vi "ResMgr-Request ExitEvent.vi"(6 "Timeout In ms (5000 ms)":i32=5000, 7 "WatchDogQ":refnum<queue>, 8 "Error In":errorcluster caption="error in (no error)") -> (0 "error out":errorcluster, 3 "CSMExit":refnum<user-event>)   [LabVIEW 2017, in "Communicable State Machine.lvlib"]
uses:
  Communicable State Machine.lvlib
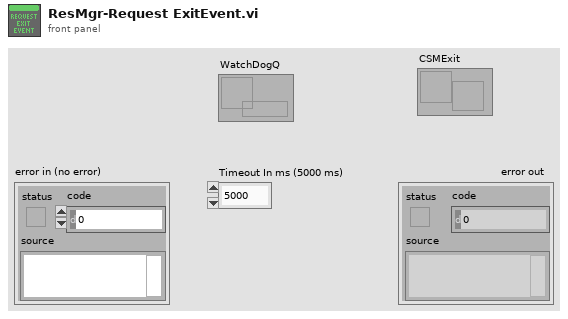
[diagram p1: front panel]
types:
  T1 = cluster{"ResType":string, "RespQ":refnum<queue>, "Parameter":string, "WatchDogQ":refnum<queue>}
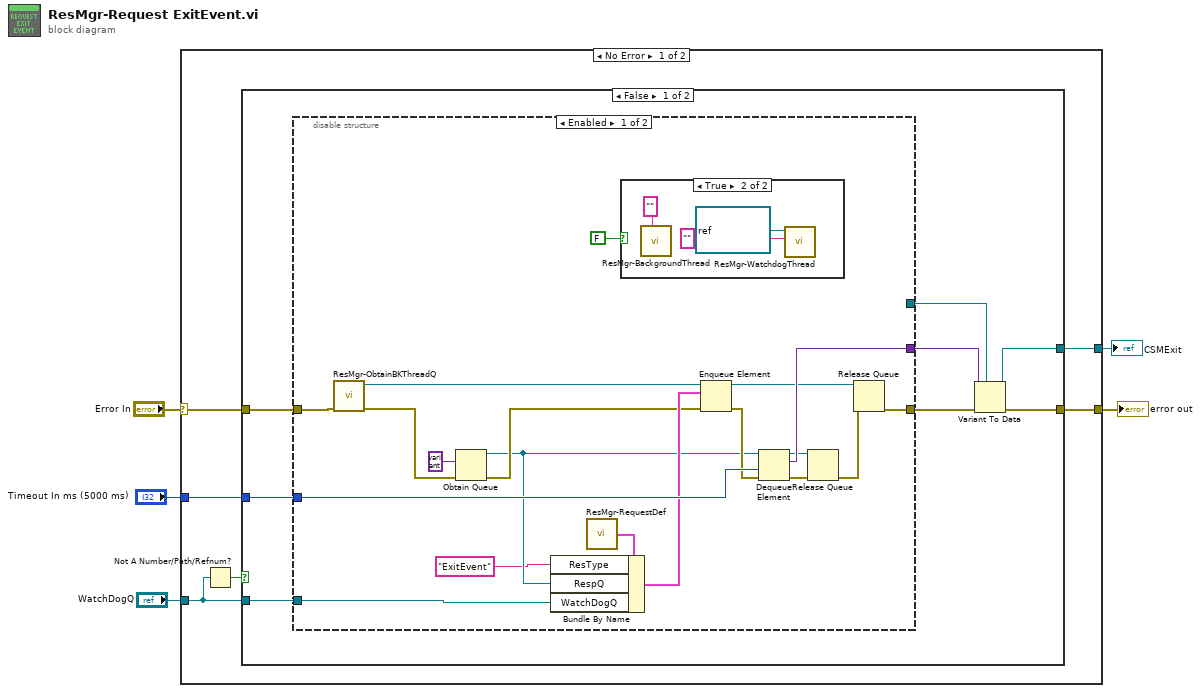
[diagram p0: block diagram]
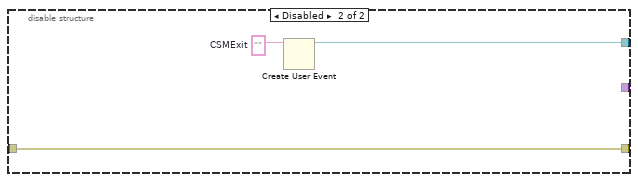
[diagram p3: hidden frame]
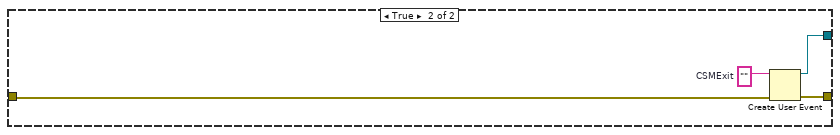
[diagram p4: hidden frame]
diagram:
  n1 = case shown="No Error" "Error In" {
    selector: "Error In" -> [w10 w49]
    tunnel: [w9 w49] -> w5
    tunnel: [w8 _] -> w1
    tunnel: "Timeout In ms (5000 ms)" -> [w11 _]
    tunnel: "WatchDogQ" -> [w7 _]
    frame No Error {
      n2 = Not A Number/Path/Refnum?(number/path/refnum=w7) -> (NaN/Path/Refnum?=w6:bool)
      n3 = case shown="False" w6 {
        tunnel: w11 -> [w18 _]
        tunnel: w10 -> [w17 w45]
        tunnel: w7 -> [w16 _]
        tunnel: [w15 w47] -> w9
        tunnel: [w12 w46] -> w8
        frame False {
          n4 = disable-structure shown="Enabled" {
            disable-tunnel: [w38 w44] -> w19
            disable-tunnel: w18 -> [w37 _]
            disable-tunnel: [w36 _] -> w14
            disable-tunnel: w17 -> [w21 w44]
            disable-tunnel: w16 -> [w25 _]
            disable-tunnel: [_ w42] -> w13
            frame Enabled {
              n5 = call "ResMgr-ObtainBKThreadQ.vi"("error in (no error)"=w21) -> ("error out"=w22:errorcluster, "ObtainBKThreadQ"=w23:refnum<queue>)  [unwired: 9 in]
              n6 = Obtain Queue(element data type=variant, error in (no error)=w22) -> (queue out=w26:refnum<queue>, error out=w34:errorcluster)  [unwired: 3 in, 1 out]
              n7 = call "ResMgr-RequestDef.vi"() -> ("ResMgr-RequestDef.ctl"=w20:T1)  [unwired: 2 in]
              n8 = Bundle By Name(cluster=w20, "ResType"="ExitEvent", "RespQ"=w26, "WatchDogQ"=w25) -> (w35:T1)
              n9 = case shown="True" FALSE {
                frame False {
                }
                frame True {
                  n10 = call "ResMgr-BackgroundThread.vi"("Name (Unnamed)"="" ("name (unnamed)")) -> ()  [unwired: 11 in]
                  n11 = call "ResMgr-WatchdogThread.vi"("From Who"="", "WatchDogQ"=refnum<queue> refnum) -> ()  [unwired: 10 in]
                }
              }
              n12 = Enqueue Element(queue=w23, element=w35, error in (no error)=w34) -> (queue out=w30:refnum<queue>, error out=w33:errorcluster)  [unwired: 1 in, 1 out]
              n13 = Dequeue Element(queue=w26, timeout in ms (-1)=w37, error in (no error)=w33) -> (queue out=w31:refnum<queue>, element=w36:variant, error out=w32:errorcluster)  [unwired: 1 out]
              n14 = Release Queue(queue=w31, error in (no error)=w32) -> (error out=w29:errorcluster)  [unwired: 1 in, 2 out]
              n15 = Release Queue(queue=w30, error in (no error)=w29) -> (error out=w38:errorcluster)  [unwired: 1 in, 2 out]
            }
            frame Disabled {
              w43 = ""  # CSMExit
              n16 = Create User Event(user event datatype=w43) -> (user event=w42:refnum<user-event>)  [unwired: 1 in, 1 out]
            }
          }
          n17 = Variant To Data(error in=w19, type=w13, Variant=w14) -> (data=w12:refnum<user-event>, error out=w15:errorcluster)
        }
        frame True {
          w48 = ""  # CSMExit
          n18 = Create User Event(user event datatype=w48, error in=w45) -> (user event=w46:refnum<user-event>, error out=w47:errorcluster)
        }
      }
    }
    frame Error {
    }
  }
  "error out" <- w5
  "CSMExit" <- w1
